vi "GET Rows.vi"(7 "Filters":T1[](array[typedef]), 8 "Error in":errorcluster caption="Error in (no error)", 11 "Table ID":u32=701) -> (0 "Error out":errorcluster, 3 "Rows Array JSON":string)   [LabVIEW 2018]
uses:
  TypeDef/FIlter.ctl
  <vilib>/JDP Science/JSONtext/Next JSON Value.vi
  <vilib>/JDP Science/JSONtext/String Subset.vi
  <vilib>/JDP Science/JSONtext/Parsing/Advance past next JSON Value (inlined COPY).vi
  <vilib>/JDP Science/JSONtext/Parsing/Advance past whitespace.vi
  <vilib>/JDP Science/JSONtext/Parsing/Advance past String.vi
  <vilib>/JDP Science/JSONtext/Parsing/Advance past Number.vi
  <vilib>/JDP Science/JSONtext/Parsing/Advance past Line Ending.vi
  Collect Param - Bool.vi
  Collect Param - String.vi
  Collect Param - Decimal.vi
  <vilib>/JDP Science/JSONtext/Parsing/Parse Full Path or Item Name.vi
  <vilib>/JDP Science/JSONtext/Parsing/Advance past Array.vi
  <vilib>/JDP Science/JSONtext/Parsing/Advance past Object.vi
  <vilib>/JDP Science/JSONtext/support/Error Cluster From Code.vi
  <vilib>/JDP Science/JSONtext/Offset/Find Item Locations by Path.vi
  <vilib>/JDP Science/JSONtext/support/Format JSON Array Text.vi
  <vilib>/httpClient/LabVIEWHTTPClient.lvlib
  <vilib>/JDP Science/JSONtext/JSONtext.lvlib
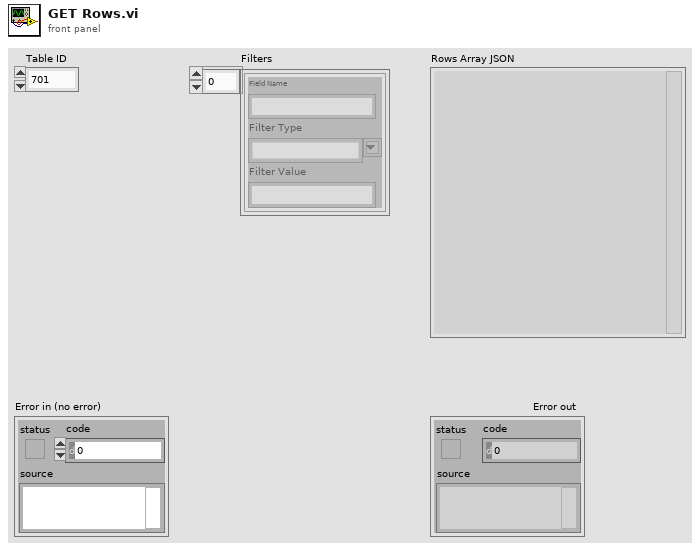
[diagram p1: front panel]
types:
  T1 = typedef "FIlter.ctl" = cluster{"Field Name":string, "Filter Type":string, "Filter Value":string}
  T2 = typedef "LabVIEWHTTPClient.lvlib/ClientHandle.ctl" = refnum<k1>
  T3 = typedef "Param.ctl" = cluster{"Param":string, "Value":string}
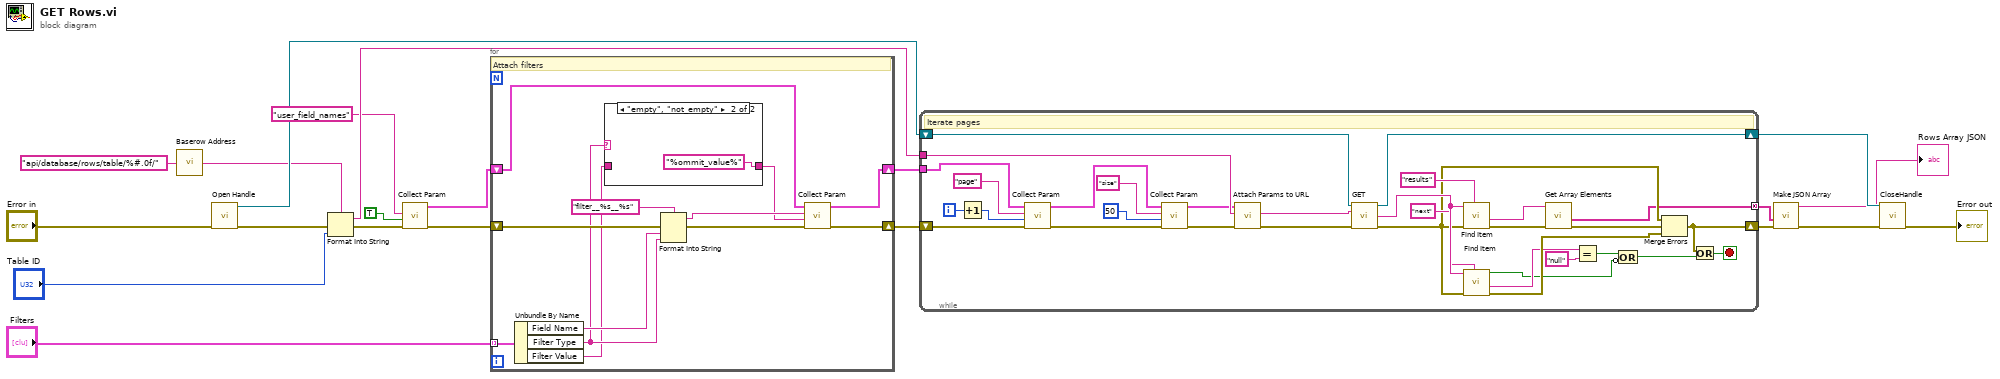
[diagram p0: block diagram]
diagram:
  n1 = call "Baserow Address.vi"("Path"="api/database/rows/table/%#.0f/" ("url")) -> ("URL + Path"=w1:string)
  n2 = call "Open Handle.vi"("error in (no error)"="Error in") -> ("error out"=w18:errorcluster, "Refnum out"=w17:T2)  [unwired: 9 in]
  n3 = Format Into String(format string=w1, error in=w18, "Table ID") -> (resulting string=w21:string, error out=w9:errorcluster)  [unwired: 1 in]
  n4 = call-poly "Collect Param.vi"("Error in"=w9, "Value"=TRUE, "Param Name"="user_field_names") -> ("Error out"=w8:errorcluster, "Params Array Out"=w11:T3[])  [unwired: 7 in]
  n5 = for {
    shift-right: [w32] -> w10
    shift-left: w11 -> [w33]
    shift-right: [w31] -> w7
    shift-left: w8 -> [w29]
    tunnel: "Filters" -> [w26] mode=indexing
    # "Attach filters"
    n6 = Unbundle By Name(w26) -> ("Field Name"=w25:string, "Filter Type"=w24:string, "Filter Value"=w22:string)
    n7 = case shown="\"empty\", \"not_empty\"" w24 {
      tunnel: [w34 "%ommit_value%" ("Filter Value")] -> w23
      tunnel: w22 -> [w34 _]
      frame Default {
      }
      frame "empty", "not_empty" {
      }
    }
    n8 = Format Into String(format string="filter__%s__%s", error in=w29, w25, w24) -> (resulting string=w27:string, error out=w28:errorcluster)  [unwired: 1 in]
    n9 = call-poly "Collect Param.vi"("Error in"=w28, "Value"=w23, "Param Name"=w27, "Params Array In"=w33) -> ("Error out"=w31:errorcluster, "Params Array Out"=w32:T3[])  [unwired: 6 in]
  }
  n10 = while {
    tunnel: [w36] -> w6 mode=concatenating
    shift-right: [w66] -> w19
    shift-left: w17 -> [w67]
    shift-right: [w62] -> w5
    shift-left: w7 -> [w43]
    tunnel: w21 -> [w51]
    tunnel: w10 -> [w45]
    i -> [w49]
    stop <- w58 stop-if-true
    # "Iterate pages"
    n11 = Increment(x=w49) -> (x+1=w48:i32)
    n12 = call-poly "Collect Param.vi"("Error in"=w43, "Value"=w48, "Param Name"="page" ("Param"), "Params Array In"=w45) -> ("Error out"=w52:errorcluster, "Params Array Out"=w55:T3[])  [unwired: 6 in]
    n13 = call-poly "Collect Param.vi"("Error in"=w52, "Value"=50, "Param Name"="size" ("Param"), "Params Array In"=w55) -> ("Error out"=w42:errorcluster, "Params Array Out"=w44:T3[])  [unwired: 6 in]
    n14 = call "Attach Params to URL.vi"("Error in"=w42, "URL"=w51, "Param array"=w44) -> ("Error out"=w46:errorcluster, "URL with params"=w47:string)  [unwired: 7 in]
    n15 = call <vilib>:"GET.vi"("client handle"=w67, "url"=w47, "error in (no error)"=w46) -> ("client handle out"=w66:T2, "body"=w64:string, "error out"=w61:errorcluster)  [unwired: 9 in, 1 out]
    n16 = call <vilib>:"Find Item.vi"("$Path or Item Name"="results", "error in (no error)"=w61, "JSON"=w64) -> ("error out"=w38:errorcluster, "<JSON>"=w39:string)  [unwired: 5 in, 2 out]
    n17 = call <vilib>:"Find Item.vi"("$Path or Item Name"="next", "error in (no error)"=w61, "JSON"=w64) -> ("error out"=w60:errorcluster, "<JSON>"=w57:string, "Found"=w40:bool)  [unwired: 5 in, 1 out]
    n18 = call <vilib>:"Get Array Elements.vi"("error in (no error)"=w38, "JSON"=w39) -> ("error out"=w37:errorcluster, "<JSON>"=w36:string[])  [unwired: 7 in, 1 out]
    n19 = Equal?(x=w57, y="null" ("x")) -> (x = y?=w59:bool)
    n20 = Compound Arithmetic op=OR(w59, invert w40) -> (w41:bool)
    n21 = Merge Errors(w61, w37, w60) -> (w62:errorcluster)
    n22 = Or(x=w62, y=w41) -> (x .or. y?=w58:bool)
  }
  n23 = call <vilib>:"Make JSON Array.vi"("error in (no error)"=w5, "JSON Elements"=w6) -> ("error out"=w4:errorcluster, "<JSON>"=→"Rows Array JSON":string)  [unwired: 8 in]
  n24 = call <vilib>:"CloseHandle.vi"("client handle"=w19, "error in (no error)"=w4) -> ("error out"=→"Error out":errorcluster)  [unwired: 13 in]
